vi "K-C.vi"(1 "Град F":dbl) -> (0 "Град C":dbl)   [LabVIEW 2020]
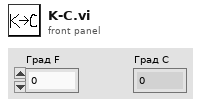
[diagram p1: front panel]
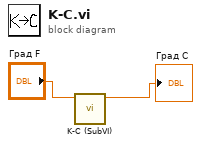
[diagram p0: block diagram]
diagram:
  n1 = call "K-C (SubVI).vi"("Град F"="Град F") -> ("Град C"=→"Град C":dbl)  [unwired: 10 in]
